vi "check File Version.vi"(10 "remote File Version Info":string, 11 "Local File Version Info":string) -> (3 "new?":bool)   [LabVIEW 2016, in "数据传输系统-04.lvlib" / "update.lvlib"]
uses:
  update.lvlib
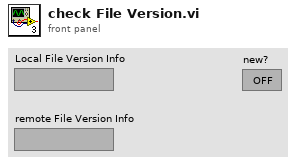
[diagram p1: front panel]
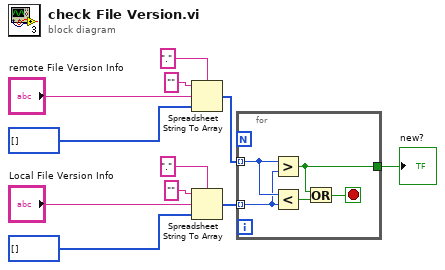
[diagram p0: block diagram]
diagram:
  n1 = Spreadsheet String To Array(delimiter (Tab)="." ("分隔符(Tab)"), format string="" ("格式字符串"), spreadsheet string="remote File Version Info", array type (2D Dbl)=i32[] []) -> (array=w10:i32[])
  n2 = Spreadsheet String To Array(delimiter (Tab)="." ("分隔符(Tab)"), format string="" ("格式字符串"), spreadsheet string="Local File Version Info", array type (2D Dbl)=i32[] []) -> (array=w11:i32[])
  n3 = for {
    tunnel: w10 -> [w16] mode=indexing
    tunnel: w11 -> [w15] mode=indexing
    tunnel: [w12] -> w3
    stop <- w13 stop-if-true
    n4 = Greater?(x=w16, y=w15) -> (0:w12:bool)
    n5 = Less?(x=w16, y=w15) -> (x < y?=w14:bool)
    n6 = Or(x=w12, y=w14) -> (x .or. y?=w13:bool)
  }
  "new?" <- w3
